vi "F5.vi"(8 "error in":errorcluster, 9 "data":u8[](array[numeric]), 10 "function":u8, 11 "device data model in":refnum<class "Standard Data Model.lvclass">) -> (0 "error out":errorcluster, 1 "data return":u8[](array[numeric]), 2 "function return":u8, 3 "device data model out":refnum<class "Standard Data Model.lvclass">)   [LabVIEW 2012, in "Standard Data Model.lvclass"]
doc: "Executes function code 5"
uses:
  Standard Data Model.lvclass
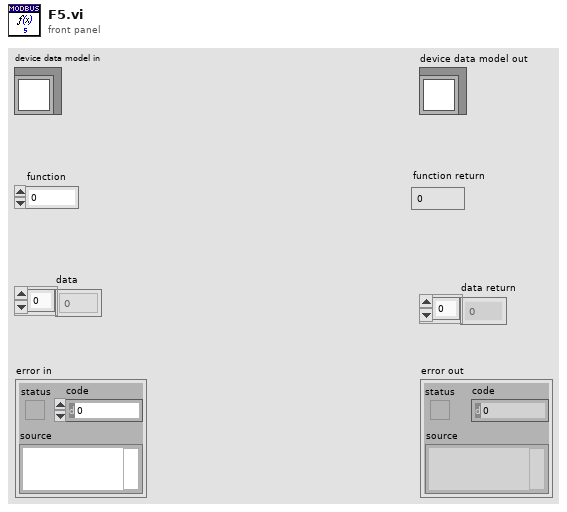
[diagram p1: front panel]
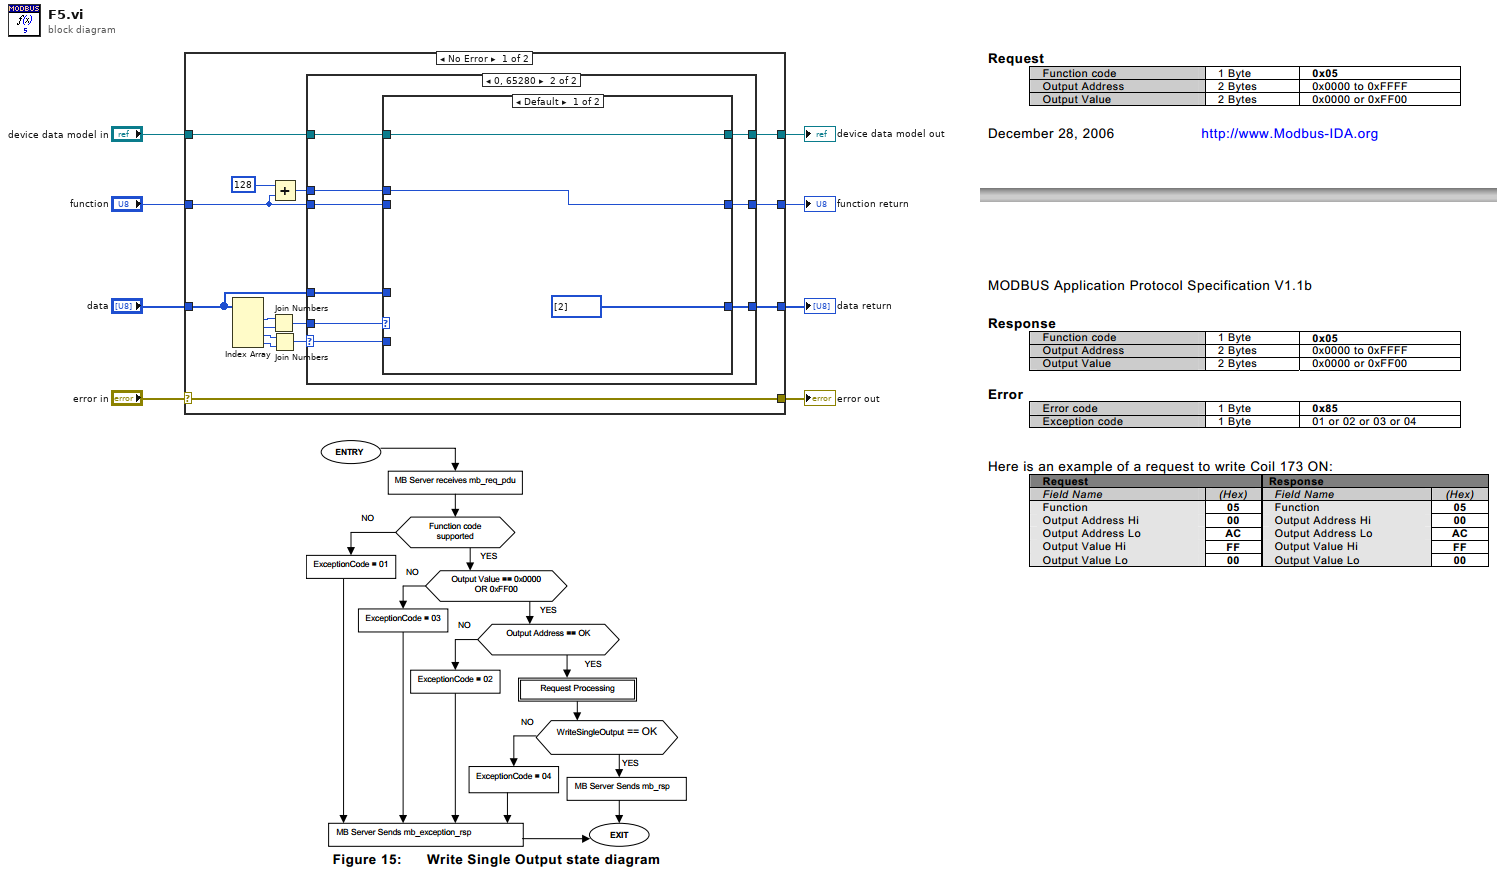
[diagram p0: block diagram]
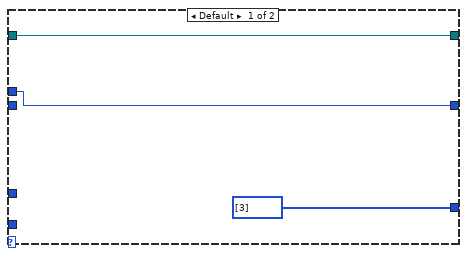
[diagram p2: hidden frame]
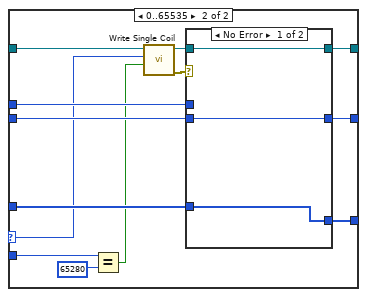
[diagram p3: hidden frame]
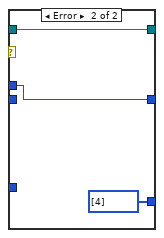
[diagram p4: hidden frame]
diagram:
  n1 = case shown="No Error" "error in" {
    selector: "error in" -> [w23 w61]
    tunnel: [w23 w61] -> w7
    tunnel: [w20 w60] -> w5
    tunnel: "device data model in" -> [w19 w60]
    tunnel: "function" -> [w16 w59]
    tunnel: "data" -> [w9 w58]
    tunnel: [w15 w59] -> w2
    tunnel: [w14 w58] -> w1
    frame No Error {
      n2 = Index Array(array=w9) -> (element #1=w21:u8, element #2=w22:u8, element #3=w12:u8, element #4=w11:u8)  [unwired: 4 in]
      n3 = Join Numbers(hi=w21, lo=w22) -> ((hi.lo)=w13:u16)
      n4 = Add(x=u8 128, y=w16) -> (x+y=w17:u8)
      n5 = Join Numbers(hi=w12, lo=w11) -> ((hi.lo)=w10:u16)
      n6 = case shown="0, 65280" w10 {
        selector: w10 -> [_ w35]
        tunnel: [w26 w34] -> w20
        tunnel: w19 -> [w26 w33]
        tunnel: w17 -> [w25 w32]
        tunnel: w16 -> [_ w30]
        tunnel: [w25 w31] -> w15
        tunnel: [u8[] [3] ("Data Return") w29] -> w14
        tunnel: w13 -> [_ w28]
        tunnel: w9 -> [_ w27]
        frame Default {
        }
        frame 0, 65280 {
          n7 = case shown="Default" w28 {
            selector: w28 -> [_ w42]
            tunnel: w35 -> [_ w40]
            tunnel: [w38 w51] -> w34
            tunnel: w33 -> [w38 w44]
            tunnel: w32 -> [w37 w50]
            tunnel: [w37 w48] -> w31
            tunnel: w30 -> [_ w49]
            tunnel: [u8[] [2] ("Data Return") w47] -> w29
            tunnel: w27 -> [_ w46]
            frame Default {
            }
            frame 0..65535 {
              n8 = Equal?(x=w40, y=u16 65280) -> (x = y?=w39:bool)
              n9 = call-dynamic "Write Single Coil.vi"("coil value"=w39, "address"=w42, "device data model in"=w44) -> ("error out"=w43:errorcluster, "device data model out"=w45:refnum<class "Standard Data Model.lvclass">)  [unwired: 7 in]
              n10 = case shown="No Error" w43 {
                tunnel: w45 -> [w54 w57]
                tunnel: [w54 w57] -> w51
                tunnel: w50 -> [_ w56]
                tunnel: w49 -> [w53 _]
                tunnel: [w53 w56] -> w48
                tunnel: [w52 u8[] [4]] -> w47
                tunnel: w46 -> [w52 _]
                frame No Error {
                }
                frame Error {
                }
              }
            }
          }
        }
      }
    }
    frame Error {
    }
  }
  "error out" <- w7
  "device data model out" <- w5
  "data return" <- w1
  "function return" <- w2
